vi "Get Signal Info from Table.vi"(11 "signal table":string[][](array[string])) -> (3 "signal parameters":T1(array[cluster]))   [LabVIEW 2022 SP3, in "Generation_Class D Amplifier_UI.lvlib"]
uses:
  Generation_Class D Amplifier_UI.lvlib
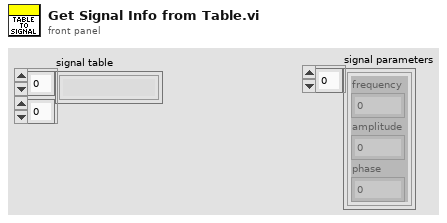
[diagram p1: front panel]
types:
  T1 = cluster{"frequency":dbl, "amplitude":dbl, "phase":dbl}[]
  T2 = cluster{"frequency":dbl, "amplitude":dbl, "phase":dbl}
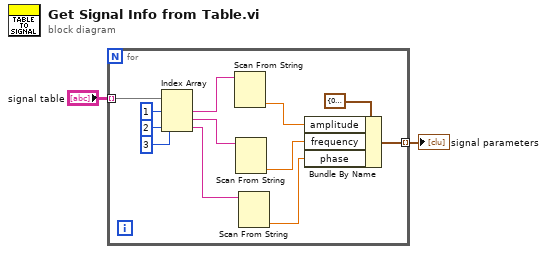
[diagram p0: block diagram]
diagram:
  n1 = for {
    tunnel: "signal table" -> [w12] mode=indexing
    tunnel: [w13] -> w1 mode=indexing
    n2 = Index Array(array=w12, index #1=1 ("index"), index #2=2 ("index"), index #3=3 ("index")) -> (element #1=w8:string, element #2=w7:string, element #3=w4:string)
    n3 = Scan From String(input string=w8) -> (output 1=w6:dbl)  [unwired: 4 in, 3 out]
    n4 = Scan From String(input string=w7) -> (output 1=w5:dbl)  [unwired: 4 in, 3 out]
    n5 = Scan From String(input string=w4) -> (output 1=w3:dbl)  [unwired: 4 in, 3 out]
    n6 = Bundle By Name(cluster=T2 {"frequency"=0.0, "amplitude"=0.0, "phase"=0.0} ("sine wave"), "amplitude"=w6, "frequency"=w5, "phase"=w3) -> (w13:T2)
  }
  "signal parameters" <- w1
